vi "Make from Library.vi"(8 "error in (no error)":errorcluster, 10 "Library Path":path, 11 "LUnit Test Suite In":refnum<class "LUnit Test Suite.lvclass">) -> (0 "error out":errorcluster, 3 "LUnit Test Suite Out":refnum<class "LUnit Test Suite.lvclass">)   [LabVIEW 2020, in "LUnit Test Suite.lvclass"]
uses:
  LUnit Test Suite.lvclass
  C:/git/astemes-lunit/source/Core/Runnable/Runnable.lvclass
  LUnit Test Case/LUnit Test Case.lvclass
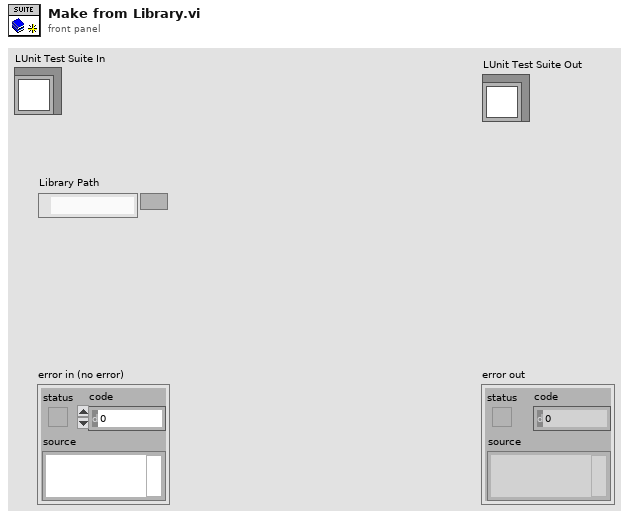
[diagram p1: front panel]
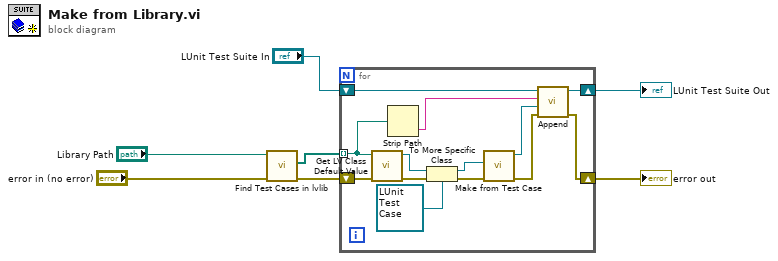
[diagram p0: block diagram]
diagram:
  n1 = call "Find Test Cases in lvlib.vi"("error in (no error)"="error in (no error)", "Project Path"="Library Path") -> ("error out"=w5:errorcluster, "Test Class paths"=w6:path[])  [unwired: 8 in]
  n2 = for {
    tunnel: w6 -> [w14] mode=indexing
    shift-right: [w18] -> w1
    shift-left: "LUnit Test Suite In" -> [w19]
    shift-right: [w12] -> w3
    shift-left: w5 -> [w20]
    n3 = call <vilib>:"Get LV Class Default Value.vi"("error in (no error)"=w20, "class path"=w14) -> ("error out"=w17:errorcluster, "object"=w16:refnum<class>)  [unwired: 8 in]
    n4 = Strip Path(path=w14) -> (name=w13:string)  [unwired: 1 out]
    n5 = To More Specific Class(target class=refnum<class "LUnit Test Case.lvclass"> refnum ("LUnit Test Case V2.lvclass"), reference=w16, error in=w17) -> (specific class reference=w9:refnum<class "LUnit Test Case.lvclass">, error out=w11:errorcluster)
    n6 = call "Make from Test Case.vi"("error in (no error)"=w11, "LUnit Test Case"=w9) -> ("error out"=w10:errorcluster, "LUnit Test Suite Out"=w8:refnum<class "LUnit Test Suite.lvclass">)  [unwired: 8 in]
    n7 = call "Append.vi"("error in (no error)"=w10, "Runnable"=w8, "Name"=w13, "LUnit Test Suite In"=w19) -> ("error out"=w12:errorcluster, "LUnit Test Suite Out"=w18:refnum<class "LUnit Test Suite.lvclass">)  [unwired: 6 in]
  }
  "error out" <- w3
  "LUnit Test Suite Out" <- w1
